vi "TCP test.vi"() -> ()   [LabVIEW 2013]
panel:
  out "bytes written":i32
  in  "String 2":string
  in  "Stop 2":bool
  in  "bytes to read":i32=512
  out "String":string
  in  "port":u16=8899
  in  "Stop":bool
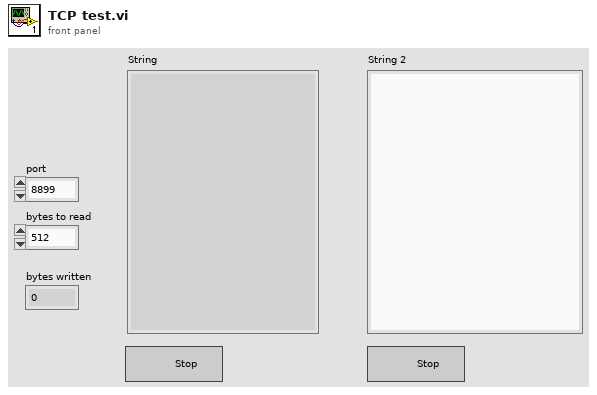
[diagram p1: front panel]
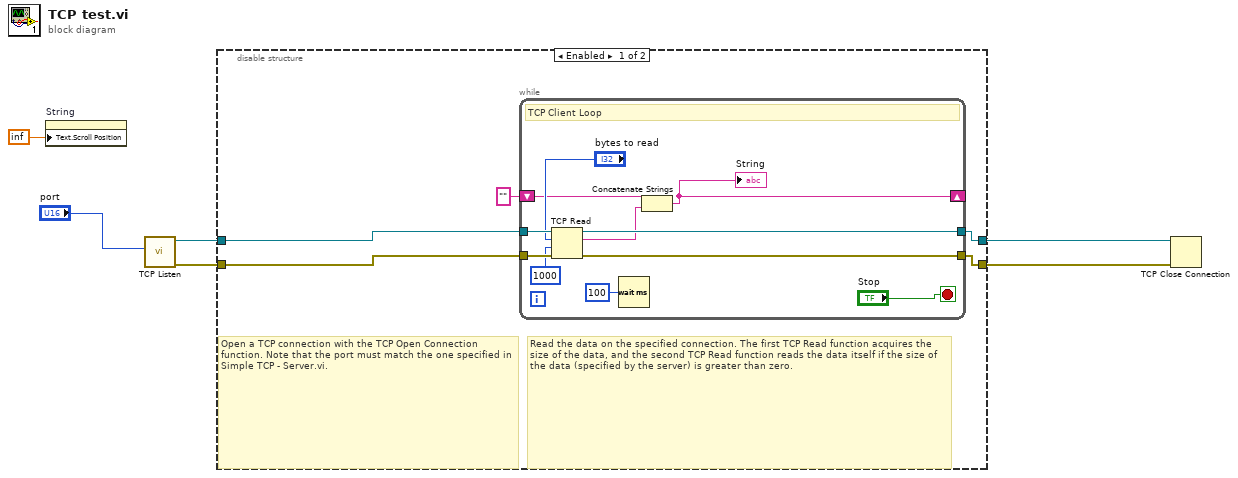
[diagram p0: block diagram]
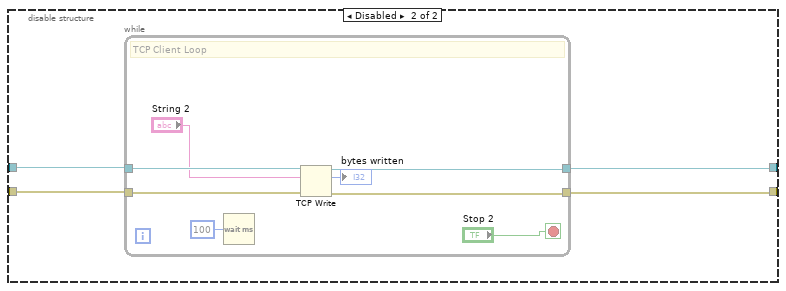
[diagram p2: hidden frame]
diagram:
  n1 = property on="String" class="Str"("Text.Scroll Position"=inf) -> ()  [unwired: 2 in, 2 out]
  n2 = call <vilib>:"TCP Listen.vi"("port"="port") -> ("error out"=w5:errorcluster, "connection ID"=w6:refnum<k5>)  [unwired: 6 in, 3 out]
  n3 = disable-structure shown="Enabled" {
    disable-tunnel: w6 -> [w11 w26]
    disable-tunnel: w5 -> [w10 w25]
    disable-tunnel: [w9 w23] -> w2
    disable-tunnel: [w8 w24] -> w3
    frame Enabled {
      # "Read the data on the specified connection. The first TCP Read function acquires the size of the data, and the second TCP Read function reads the data itself if the size of the data (specified by the server) is greater than zero."
      # "Open a TCP connection with the TCP Open Connection function. Note that the port must match the one specified in Simple TCP - Server.vi."
      n4 = while {
        tunnel: w10 -> [w21]
        tunnel: w11 -> [w22]
        tunnel: [w17] -> w9
        tunnel: [w16] -> w8
        shift-right: [w12] -> _
        shift-left: "" -> [w13]
        stop <- "Stop" stop-if-true
        # "TCP Client Loop"
        n5 = TCP Read(connection ID=w22, bytes to read="bytes to read", error in (no error)=w21, 9:1000 ("timeout ms (25000)")) -> (connection ID out=w16:refnum<k5>, data out=w14:string, error out=w17:errorcluster)  [unwired: 1 in]
        n6 = Wait (ms)(milliseconds to wait=u32 100) -> ()  [unwired: 1 out]
        n7 = Concatenate Strings(w13, w14) -> (w12:string)
        "String" <- w12
      }
    }
    frame Disabled {
      n8 = while {
        tunnel: w25 -> [w31]
        tunnel: w26 -> [w32]
        tunnel: [w30] -> w23
        tunnel: [w29] -> w24
        stop <- "Stop 2" stop-if-true
        # "TCP Client Loop"
        n9 = Wait (ms)(milliseconds to wait=u32 100) -> ()  [unwired: 1 out]
        n10 = TCP Write(connection ID=w32, data in="String 2", error in (no error)=w31) -> (connection ID out=w29:refnum<k5>, bytes written=→"bytes written":i32, error out=w30:errorcluster)  [unwired: 1 in]
      }
    }
  }
  n11 = TCP Close Connection(connection ID=w3, error in (no error)=w2) -> ()  [unwired: 1 in, 2 out]
